vi "Using Analysis tools (Waveform data type).vi"() -> ()   [LabVIEW 2020]
uses:
  <vilib>/DAQmx/read.llb/DAQmx Read (Analog Wfm 1Chan NSamp).vi
  <vilib>/DAQmx/miscellaneous.llb/DAQmx Fill In Error Info.vi
  <vilib>/measure/mascope.llb/Amplitude and Levels 1 chan.vi
  <vilib>/DAQmx/configure/timing.llb/DAQmx Timing (Sample Clock).vi
  <vilib>/DAQmx/create/channels.llb/DAQmx Create Channel (AI-Temperature-Thermocouple).vi
  <resource>/objmgr/daqmx.rc
  <vilib>/measure/NI_MAPro.lvlib
panel:
  out "max value":dbl
  out "Acquired Signal":waveform(dbl)(graph)
  in  "Stop":bool
  out "Actual Sample Rate (Hz)":dbl
  in  "Number of Samples":i32=1000
  in  "Desired Sample Rate (Hz)":dbl=1000.0
  in  "Physical Channel":tag="PCI-6221/ai0"
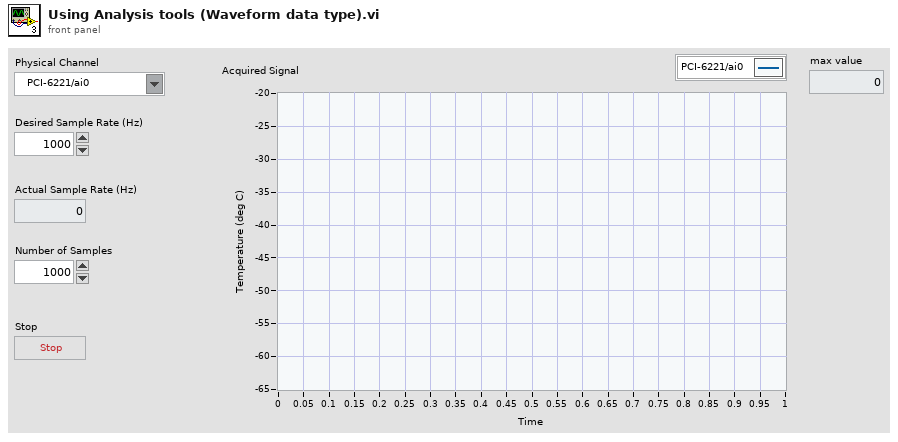
[diagram p1: front panel]
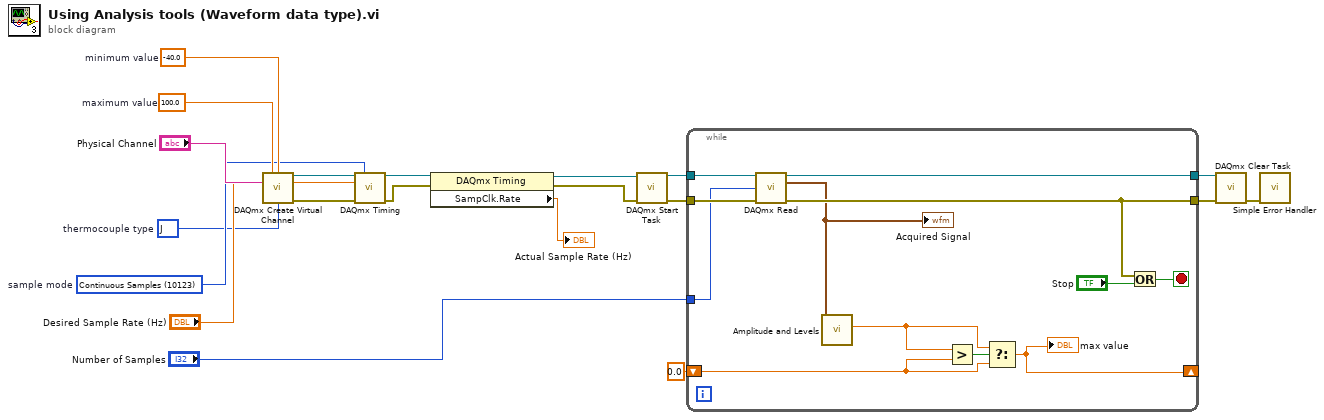
[diagram p0: block diagram]
diagram:
  w2 = 10072 items=["J"=10072, "K"=10073, "N"=10077, "R"=10082, "S"=10085, "T"=10086, "B"=10047, "E"=10055]  # thermocouple type
  w17 = 10123 items=["Finite Samples"=10178, "Continuous Samples"=10123, "Hardware Timed Single Point"=12522]  # sample mode
  w19 = 100.0  # maximum value
  w20 = -40.0  # minimum value
  n1 = call-poly <vilib>:"DAQmx Create Virtual Channel.vi"("maximum value"=w19, "minimum value"=w20, "physical channels"="Physical Channel", "thermocouple type"=w2) -> ("task out"=w15:refnum<k21>, "error out"=w14:errorcluster)  [unwired: 10 in]
  n2 = call-poly <vilib>:"DAQmx Timing.vi"("task/channels in"=w15, "sample mode"=w17, "rate"="Desired Sample Rate (Hz)", "error in"=w14) -> ("task out"=w13:refnum<k21>, "error out"=w12:errorcluster)  [unwired: 10 in]
  n3 = property class="DAQmx Timing"(reference=w13, error in=w12) -> (reference out=w10:refnum<k21>, error out=w9:errorcluster, "SampClk.Rate"=→"Actual Sample Rate (Hz)":dbl)
  n4 = call <vilib>:"DAQmx Start Task.vi"("task/channels in"=w10, "error in"=w9) -> ("task out"=w8:refnum<k21>, "error out"=w7:errorcluster)  [unwired: 12 in]
  n5 = while {
    tunnel: w8 -> [w32]
    tunnel: w7 -> [w31]
    tunnel: "Number of Samples" -> [w30]
    tunnel: [w29] -> w5
    tunnel: [w28] -> w4
    shift-right: [w22] -> _
    shift-left: 0.0 ("high state level") -> [w21]
    stop <- w26 stop-if-true
    n6 = call-poly <vilib>:"DAQmx Read.vi"("task/channels in"=w32, "number of samples per channel"=w30, "error in"=w31) -> ("task out"=w29:refnum<k21>, "data"=w25:waveform(dbl), "error out"=w28:errorcluster)  [unwired: 10 in]
    "Acquired Signal" <- w25
    n7 = call-poly <vilib>:"Amplitude and Levels.vi"("signal in"=w25) -> ("high state level"=w23:dbl)  [unwired: 7 in, 3 out]
    n8 = Greater?(x=w23, y=w21) -> (0:w24:bool)
    n9 = Select(t=w23, s=w24, f=w21) -> (s? t:f=w22:dbl)
    "max value" <- w22
    n10 = Or(x=w28, y="Stop") -> (x .or. y?=w26:bool)
  }
  n11 = call <vilib>:"DAQmx Clear Task.vi"("task in"=w5, "error in"=w4) -> ("error out"=w3:errorcluster)  [unwired: 13 in]
  n12 = call <vilib>:"Simple Error Handler.vi"("error in (no error)"=w3) -> ()  [unwired: 4 in, 5 out]
